vi "set_dac_polarity.vi"(8 "error in (no error)":errorcluster, 9 "DAC polarity":string, 10 "DAC number":u8, 11 "VISA resource name":refnum<visa-resource-name>) -> (0 "error out":errorcluster, 3 "VISA resource name out":refnum<visa-resource-name>)   [LabVIEW 2018]
doc: "Update the type of an output.\n\nOutputs can be normally open or normally closed."
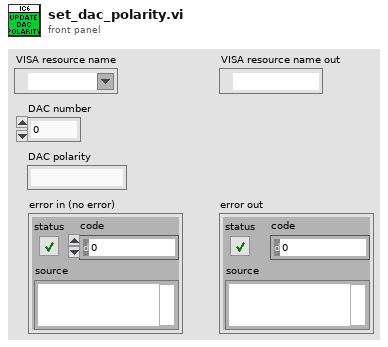
[diagram p1: front panel]
types:
  T1 = enum16{"Source", "General", "Input name", "Process name", "Logic", "Material", "Material name", "Output name", "Process", "Sensor", "Output type", "User message", "Layer", ""}
  T2 = enum16{"Hello", "Query", "Remote action", "Status", "Update"}
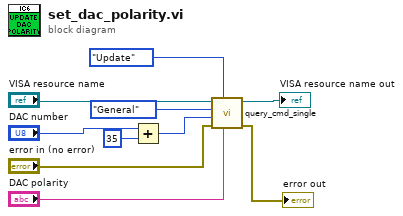
[diagram p0: block diagram]
diagram:
  n1 = Add(x="DAC number", y=u8 35) -> (x+y=w1:u8)
  n2 = call "query_cmd_single.vi"("Parameter"="DAC polarity", "Command group"=T2."Update", "error in (no error)"="error in (no error)", "Command ID"=w1, "Command subgroup"=T1."General", "VISA resource name"="VISA resource name") -> ("error out"=→"error out":errorcluster, "VISA resource name out"=→"VISA resource name out":refnum<visa-resource-name>)  [unwired: 1 in, 3 out]
